vi "Flatten Value.vi"(0 "String In":refnum<class "String.lvclass">, 11 "Error In":errorcluster) -> (4 "String Out":refnum<class "String.lvclass">, 8 "Value":string, 15 "Error Out":errorcluster)   [LabVIEW 2016, in "String.lvclass"]
uses:
  String.lvclass
  String.lvclass/String.ctl
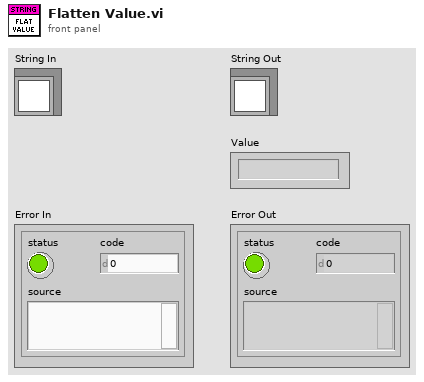
[diagram p1: front panel]
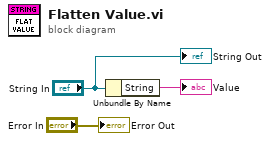
[diagram p0: block diagram]
diagram:
  n1 = Unbundle By Name("String In") -> ("String"=→"Value":string)
  "String Out" <- "String In"
  "Error Out" <- "Error In"
